vi "EspacioEstados.vi"(0 "entrada planta":dbl, 8 "salida planta":dbl, 11 "xk +1":T1=[[0.0], [0.0]]) -> (1 "Perturbacion":dbl, 3 "xk":T1)   [LabVIEW 2018]
uses:
  <vilib>/Analysis/Matrix/Datatypes/RealMatrix.ctl
  <vilib>/Analysis/Matrix/Numeric/Conversions/Array To Matrix - RA.vi
  <vilib>/Analysis/Matrix/Numeric/Conversions/Array To Matrix - RA2.vi
  <vilib>/Analysis/Matrix/Numeric/Multiply/Multiply - RM,RM.vi
  <vilib>/Analysis/Matrix/Numeric/Add/Add - RM,RM.vi
  <vilib>/Analysis/Matrix/NI_Matrix.lvlib
panel:
  out "A + B":T1
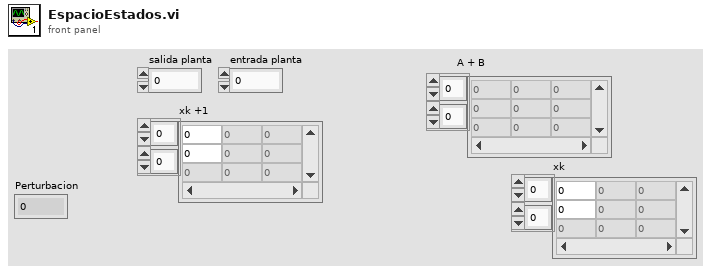
[diagram p1: front panel]
types:
  T1 = typedef "NI_Matrix.lvlib/RealMatrix.ctl" = dbl[][]
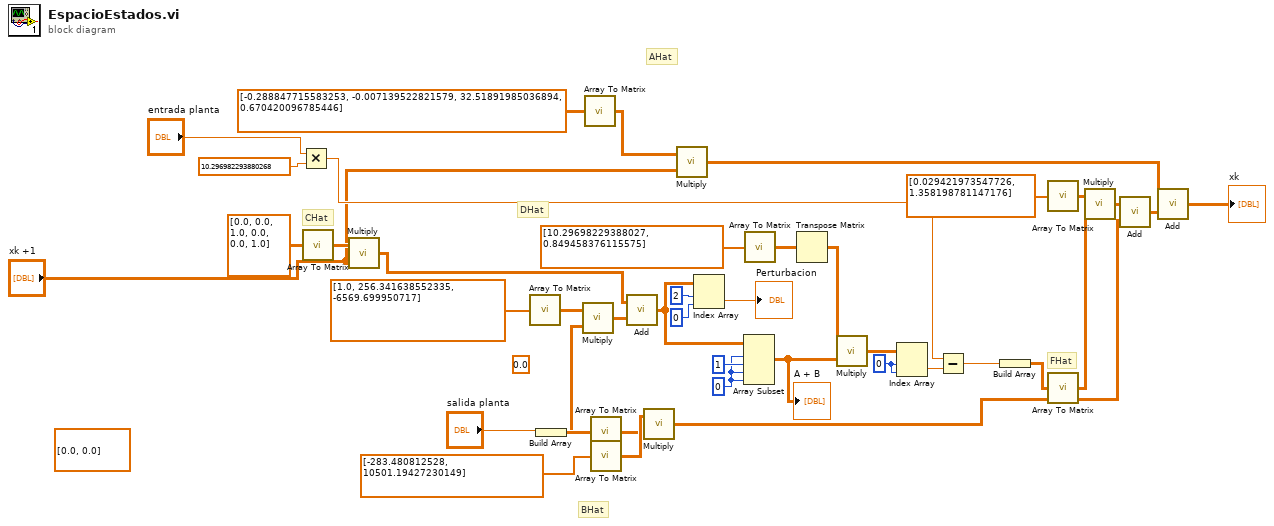
[diagram p0: block diagram]
diagram:
  (unwired) 0.0
  (unwired) T1 [[0.0], [0.0]] ("A + B")
  w35 = 0 ("index (row)")
  w37 = 0 ("row 1")
  # "DHat"
  # "CHat"
  # "FHat"
  # "AHat"
  # "BHat"
  n1 = Multiply ("Multiply.vi")(x="entrada planta", y=10.296982293880268) -> (x*y=w9:dbl)
  n2 = call-poly <vilib>:"Array To Matrix.vi"("Real 2D Array"=dbl[][] [[0.0, 0.0], [1.0, 0.0], [0.0, 1.0]]) -> ("Real Matrix"=w17:T1)
  n3 = call-poly <vilib>:"Multiply.vi"("Real Matrix B"="xk +1", "Real Matrix A"=w17) -> ("A * B"=w16:T1)
  n4 = call-poly <vilib>:"Array To Matrix.vi"("Real 1D Array"=dbl[] [1.0, 256.341638552335, -6569.699950717] ("element")) -> ("Real Matrix (Column Vector)"=w27:T1)
  n5 = Build Array("salida planta") -> (w39:T1)
  n6 = call-poly <vilib>:"Array To Matrix.vi"("Real 2D Array"=dbl[][] [[-0.288847715583253, -0.007139522821579], [32.51891985036894, 0.670420096785446]] ("element")) -> ("Real Matrix"=w26:T1)
  n7 = call-poly <vilib>:"Array To Matrix.vi"("Real 2D Array"=w39) -> ("Real Matrix"=w20:T1)
  n8 = call-poly <vilib>:"Multiply.vi"("Real Matrix B"=w20, "Real Matrix A"=w27) -> ("A * B"=w18:T1)
  n9 = call-poly <vilib>:"Array To Matrix.vi"("Real 1D Array"=dbl[] [-283.480812528, 10501.19427230149] ("element")) -> ("Real Matrix (Column Vector)"=w21:T1)
  n10 = call-poly <vilib>:"Add.vi"("Real Matrix B"=w18, "Real Matrix A"=w16) -> ("A + B"=w8:T1)
  n11 = call-poly <vilib>:"Multiply.vi"("Real Matrix B"=w20, "Real Matrix A"=w21) -> ("A * B"=w19:T1)
  n12 = call-poly <vilib>:"Multiply.vi"("Real Matrix B"="xk +1", "Real Matrix A"=w26) -> ("A * B"=w25:T1)
  n13 = Index Array(array=w8, index (row)=2, index (col)=0) -> (element=→"Perturbacion":dbl)
  n14 = Array Subset(array=w8, index (row)=w37, length (row)=1 ("row N"), index (col)=w37, length (col)=w37) -> (w14:T1)
  "A + B" <- w14
  n15 = call-poly <vilib>:"Array To Matrix.vi"("Real 1D Array"=dbl[] [10.29698229388027, 0.849458376115575] ("element")) -> ("Real Matrix (Column Vector)"=w36:T1)
  n16 = Transpose Matrix(1:w36) -> (0:w15:T1)
  n17 = call-poly <vilib>:"Multiply.vi"("Real Matrix B"=w14, "Real Matrix A"=w15) -> ("A * B"=w13:T1)
  n18 = Index Array(array=w13, index (row)=w35, index (col)=w35) -> (element=w11:dbl)
  n19 = Subtract(x=w9, y=w11) -> (x-y=w33:dbl)
  n20 = Build Array(w33) -> (w40:T1)
  n21 = call-poly <vilib>:"Array To Matrix.vi"("Real 1D Array"=dbl[] [0.029421973547726, 1.358198781147176] ("element")) -> ("Real Matrix (Column Vector)"=w24:T1)
  n22 = call-poly <vilib>:"Array To Matrix.vi"("Real 2D Array"=w40) -> ("Real Matrix"=w23:T1)
  n23 = call-poly <vilib>:"Multiply.vi"("Real Matrix B"=w23, "Real Matrix A"=w24) -> ("A * B"=w22:T1)
  n24 = call-poly <vilib>:"Add.vi"("Real Matrix B"=w19, "Real Matrix A"=w22) -> ("A + B"=w34:T1)
  n25 = call-poly <vilib>:"Add.vi"("Real Matrix B"=w34, "Real Matrix A"=w25) -> ("A + B"=→"xk":T1)
